vi "IntensityTemperature.vi"() -> ()   [LabVIEW 2020]
panel:
  in  "IntTemp":dbl[][](array[numeric])=[[100.0, 100.0, 100.0, 100.0, 100.0, 100.0, 100.0, 100.0, 100.0, 100.0, 100.0, 100.0, 100.0, 100.0, 100.0, 100.0], [-300.0, -300.0, -300.0, -300.0, -300.0, -300.0, -300.0, -300.0, -300.0, -300.0, -300.0, -300.0, -300.0, -300.0, -300.0, -300.0]]
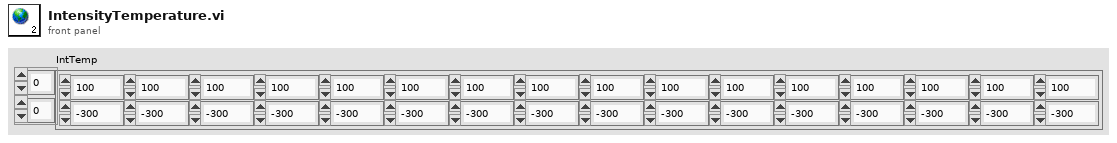
[diagram p1: front panel]
diagram:
